vi "Do.vi"(8 "error in (no error)":errorcluster, 10 "Actor in":refnum<class "Actor.lvclass">, 11 "UpdateChart":refnum<class "UpdateChart Msg.lvclass">) -> (0 "error out":errorcluster, 2 "Actor out":refnum<class "Actor.lvclass">)   [LabVIEW 2018, in "TestViewables.lvlib" / "UpdateChart Msg.lvclass"]
doc: "(<B>Filename</B>: Actor Framework.lvlib:Message.lvclass:Do.vi)\n\nDefines what a message does when it is received by an actor. Generally, a message instructs an actor to invoke one of its methods. By default, this method does nothing. A child class must override it to define behavior. Create a child class by using the Actor Framework Message Maker dialog box.\n\n<License>\nCopyright © 2017 Composed Systems, LLC | All rights reserved\nwww.composed.io\n\nAuthor: Ethan Stern <ethan.stern@composed.io>\n\nThis software is provided \"AS IS\" WITHOUT WARRANTIES, either express or implied, AND IS FOR EDUCATIONAL PURPOSES ONLY.\n</License>"
uses:
  UpdateChart Msg.lvclass
  MultiSubscriber/MultiSubscriber.lvclass
  <vilib>/ActorFramework/Actor/Actor.lvclass
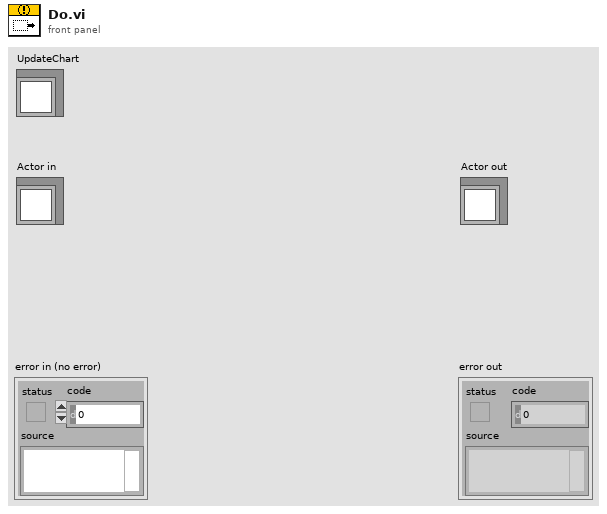
[diagram p1: front panel]
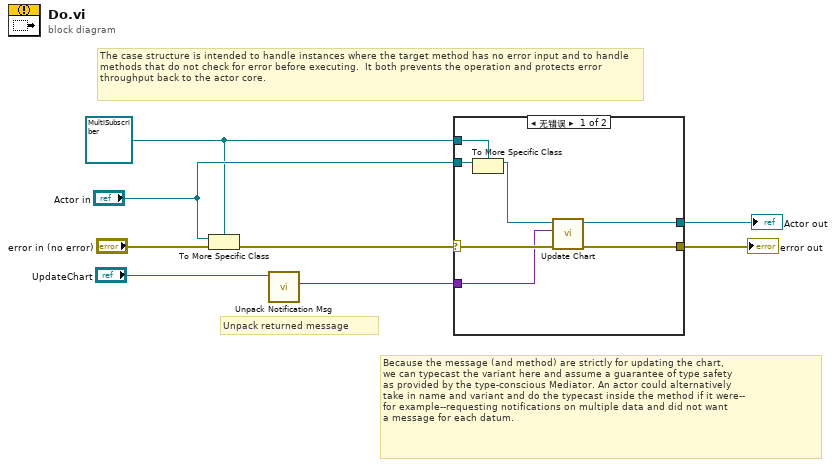
[diagram p0: block diagram]
diagram:
  w3 = refnum<class "MultiSubscriber.lvclass"> refnum ("TestActors.lvlib:MultiSubscriber.lvclass")
  # "Unpack returned message"
  # "Because the message (and method) are strictly for updating the chart,\nwe can typecast the variant here and assume a guarantee of type safety\nas provided by the type-conscious Mediator. An actor could alternatively\ntake in name and variant and do the typecast inside the method if it were--\nfor example--requesting notifications on multiple data and did not want\na message for each datum."
  # "The case structure is intended to handle instances where the target method has no error input and to handle methods that do not check for error before executing.  It both prevents the operation and protects error throughput back to the actor core."
  n1 = To More Specific Class(target class=w3, reference="Actor in", error in="error in (no error)") -> (error out=w8:errorcluster)  [unwired: 1 out]
  n2 = call-dynamic "Unpack Notification Msg.vi"("Notification Msg"="UpdateChart") -> ("Value"=w1:variant)  [unwired: 8 in, 2 out]
  n3 = case shown="无错误" w8 {
    selector: w8 -> [w13 w17]
    tunnel: [w12 w17] -> w6
    tunnel: [w10 w16] -> w5
    tunnel: "Actor in" -> [w15 w16]
    tunnel: w3 -> [w14 _]
    tunnel: w1 -> [w9 _]
    frame No Error {
      n4 = To More Specific Class(target class=w14, reference=w15) -> (specific class reference=w11:refnum<class "MultiSubscriber.lvclass">)  [unwired: 1 in, 1 out]
      n5 = call "Update Chart.vi"("error in (no error)"=w13, "Variant"=w9, "MultiSubscriber in"=w11) -> ("error out"=w12:errorcluster, "MultiSubscriber out"=w10:refnum<class "MultiSubscriber.lvclass">)  [unwired: 7 in]
    }
    frame Error {
      # "If type check fails, pass the original object out again."
    }
  }
  "error out" <- w6
  "Actor out" <- w5
